vi "MSGR Get Unique Q.vi"(8 "error in (no error)":errorcluster) -> (0 "error out":errorcluster, 2 "MSGR Q name":T3, 3 "MSG Q":T2)   [LabVIEW 2018]
doc: "$Author::Richard Jennings $\n$Rev:: $\n$Date:: May, 2008 $\n\nOVERVIEW:\nReentrant VI to receive messages via a MSGR Q. If the Q does not exist this VI will create it, then wait for data.\n\nINPUTS (Controls):\n<name> - <short description of each control wired to connector pane>\n\nOUTPUTS (Indicators):\n<name> - <short description of each indicator wired to connector pane>\n\nCopyright 2008 - 2017 Jennings Embedded Servies. All rights reserved.\nAuthor makes no warranties or guarantees related to performance of the software.\nUSE AT YOUR OWN RISK\nwww.jembedded.com\n\n\n\nMIT License\n\nCopyright (c) 2020 RichardLGP5\n\nPermission is hereby granted, free of charge, to any person obtaining a copy\nof this software and associated documentation files (the \"Software\"), to deal\nin the Software without restriction, including without limitation the rights\nto use, copy, modify, merge, publish, distribute, sublicense, and/or sell\ncopies of the Software, and to permit persons to whom the Software is\nfurnished to do so, subject to the following conditions:\n\nThe above copyright notice and this permission notice shall be included in all\ncopies or substantial portions of the Software.\n\nTHE SOFTWARE IS PROVIDED \"AS IS\", WITHOUT WARRANTY OF ANY KIND, EXPRESS OR\nIMPLIED, INCLUDING BUT NOT LIMITED TO THE WARRANTIES OF MERCHANTABILITY,\nFITNESS FOR A PARTICULAR PURPOSE AND NONINFRINGEMENT. IN NO EVENT SHALL THE\nAUTHORS OR COPYRIGHT HOLDERS BE LIABLE FOR ANY CLAIM, DAMAGES OR OTHER\nLIABILITY, WHETHER IN AN ACTION OF CONTRACT, TORT OR OTHERWISE, ARISING FROM,\nOUT OF OR IN CONNECTION WITH THE SOFTWARE OR THE USE OR OTHER DEALINGS IN THE\nSOFTWARE."
uses:
  MSGR Q Name TypeDef.ctl
  MSGR Q Ref TypeDef.ctl
  MSGR Q Data TypeDef.ctl
  MSGR Registry Control TypeDef.ctl
panel:
  in  "MSGR Q Data TypeDef":T1
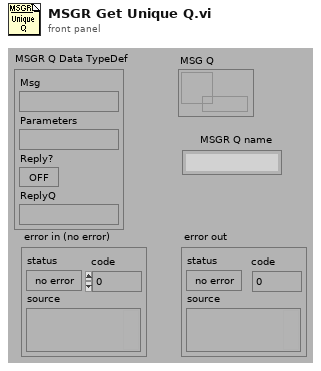
[diagram p1: front panel]
types:
  T1 = typedef "MSGR Q Data TypeDef.ctl" = cluster{"Msg":string, "Parameters":string, "Reply?":bool, "ReplyQ":string}
  T2 = typedef "MSGR Q Ref TypeDef.ctl" = refnum<queue>
  T3 = typedef "MSGR Q Name TypeDef.ctl" = string
  T4 = typedef "MSGR Registry Control TypeDef.ctl" = enum16{"reset", "register", "get data", "set data", "unregister", "test", "get objects"}
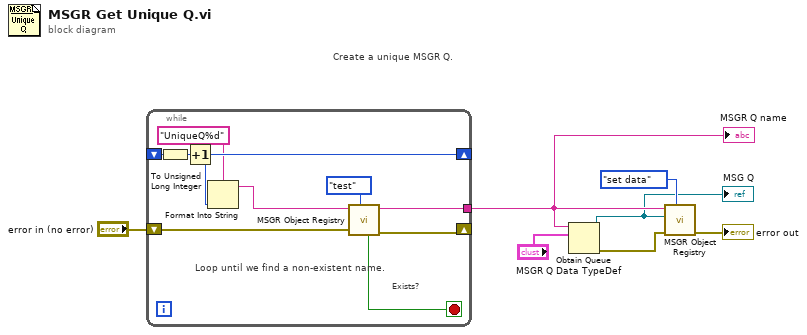
[diagram p0: block diagram]
diagram:
  # "Create a unique MSGR Q."
  n1 = while {
    tunnel: [w17] -> w2
    shift-right: [w15] -> _
    shift-left: _ -> [w14]
    shift-right: [w8] -> _
    shift-left: "error in (no error)" -> [w9]
    stop <- w10 stop-if-true
    # "Loop until we find a non-existent name."
    # "Exists?"
    n2 = To Unsigned Long Integer(number=w14) -> (unsigned 32bit integer=w13:u32)
    n3 = Increment(x=w13) -> (x+1=w15:u32)
    n4 = Format Into String(format string="UniqueQ%d", w15) -> (resulting string=w11:string)  [unwired: 2 in, 1 out]
    n5 = call "MSGR Object Registry.vi"("function (get data)"=MSGR_Registry_Control_TypeDef."test", "error in (no error)"=w9, "MSGR Q name"=w11) -> ("error out"=w8:errorcluster, "MSGR Q name"=w17:T3, "valid index?"=w10:bool)  [unwired: 4 in, 2 out]
  }
  "MSGR Q name" <- w2
  n6 = Obtain Queue(name (unnamed)=w2, element data type="MSGR Q Data TypeDef") -> (queue out=w1:refnum<queue>, error out=w4:errorcluster)  [unwired: 3 in, 1 out]
  "MSG Q" <- w1
  n7 = call "MSGR Object Registry.vi"("function (get data)"=MSGR_Registry_Control_TypeDef."set data", "error in (no error)"=w4, "MSGR Q"=w1, "MSGR Q name"=w2) -> ("error out"=→"error out":errorcluster)  [unwired: 3 in, 4 out]
